vi "Main_Motor_EMG_Control.vi"(0 "VISA Refnum in":refnum<visa-resource-name>, 1 "Motor speed":dbl format="%#_13g", 5 "EMG control":T1(ring)=enum."Biceps contracted", 7 "ID motors":i32[](array[numeric])=[41, 42, 43, 44, 45, 46, 47], 9 "Address current load":u8[](array[numeric])=[108, 110, 112, 114, 116, 118, 120], 11 "error in (no error)":errorcluster, 12 "Old positions":dbl[](array[numeric]), 13 "Old Current (mA)":dbl[](array[numeric])) -> (4 "VISA Refnum out":refnum<visa-resource-name>, 6 "Actual positions":dbl[](array[numeric]), 8 "Current (mA)":dbl[](array[numeric]), 15 "error out":errorcluster)   [LabVIEW 2015]
uses:
  <instrlib>/Dynamixel Motor/Dynamixel Motor.lvlib
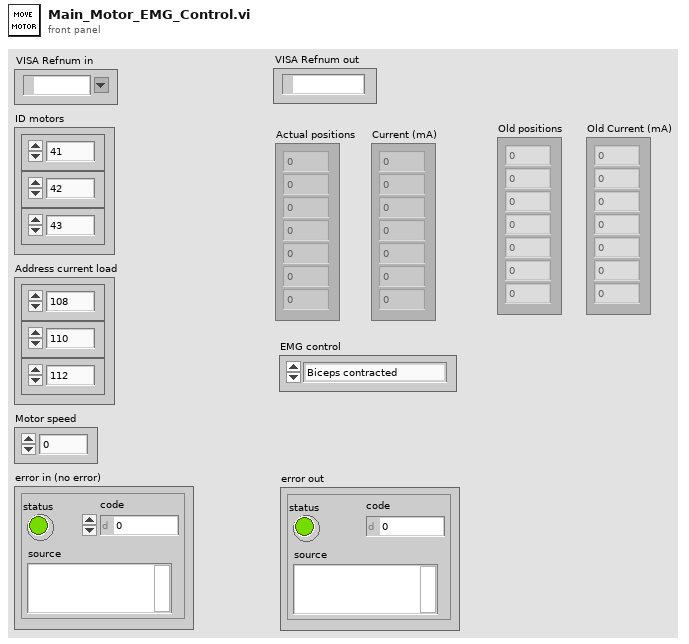
[diagram p1: front panel]
types:
  T1 = enum16{"Biceps contracted M3", "Biceps contracted", "Triceps contracted M3", "Triceps contracted"}
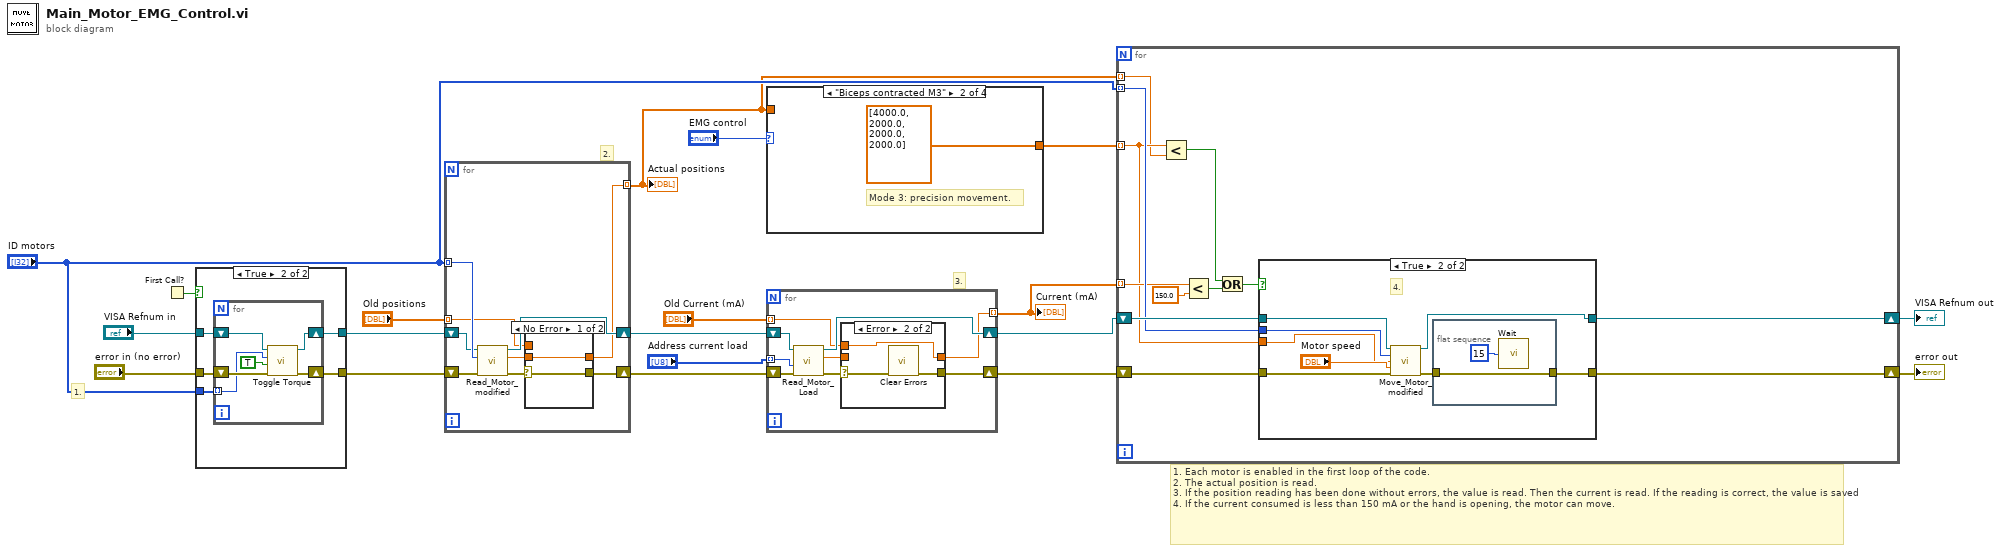
[diagram p0: block diagram]
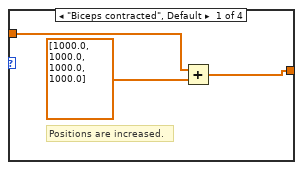
[diagram p2: hidden frame]
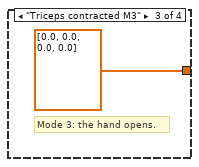
[diagram p3: hidden frame]
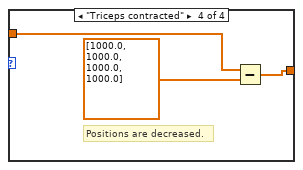
[diagram p4: hidden frame]
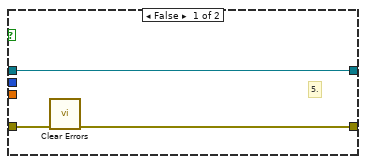
[diagram p5: hidden frame]
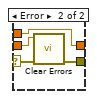
[diagram p7: hidden frame]
diagram:
  # "3."
  # "2."
  # "1."
  # "1. Each motor is enabled in the first loop of the code.\n2. The actual position is read.\n3. If the position reading has been done without errors, the value is read. Then the current is read. If the reading is correct, the value is saved\n4. If the current consumed is less than 150 mA or the hand is opening, the motor can move."
  n1 = First Call?() -> (First Call?: T/F=w10:bool)
  n2 = case shown="True" w10 {
    tunnel: "VISA Refnum in" -> [w20 w26]
    tunnel: "error in (no error)" -> [w21 w25]
    tunnel: [w20 w24] -> w13
    tunnel: [w21 w23] -> w14
    tunnel: "ID motors" -> [_ w22]
    frame False {
    }
    frame True {
      n3 = for {
        shift-right: [w30] -> w24
        shift-left: w26 -> [w31]
        shift-right: [w28] -> w23
        shift-left: w25 -> [w29]
        tunnel: w22 -> [w27] mode=indexing
        n4 = call <instrlib>:"Toggle Torque.vi"("error in (no error)"=w29, "Toggle torque (OFF)"=TRUE, "Motor ID (0)"=w27, "VISA resource name"=w31) -> ("error out"=w28:errorcluster, "VISA resource name out"=w30:refnum<visa-resource-name>)  [unwired: 6 in]
      }
    }
  }
  n5 = for {
    tunnel: "ID motors" -> [w41] mode=indexing
    shift-right: [w33] -> w16
    shift-left: w14 -> [w40]
    shift-right: [w38] -> w15
    shift-left: w13 -> [w39]
    tunnel: [w36] -> w4 mode=indexing
    tunnel: "Old positions" -> [w34] mode=indexing
    n6 = call "Read_Motor_modified.vi"("error in (no error)"=w40, "Motor ID (0)"=w41, "VISA Refnum in"=w39) -> ("error out"=w37:errorcluster, "Position"=w35:dbl, "VISA Refnum out"=w38:refnum<visa-resource-name>)  [unwired: 6 in]
    n7 = case shown="No Error" w37 {
      selector: w37 -> [w42 w45]
      tunnel: [w43 w47] -> w36
      tunnel: w35 -> [w43 w46]
      tunnel: w34 -> [_ w47]
      tunnel: [w42 w44] -> w33
      frame No Error {
      }
      frame Error {
        n8 = call <vilib>:"Clear Errors.vi"("error in (no error)"=w45, "specific error code to clear (0: all)"=w46) -> ("error out"=w44:errorcluster)  [unwired: 4 in, 1 out]
      }
    }
  }
  "Actual positions" <- w4
  n9 = case shown="\"Biceps contracted M3\"" "EMG control" {
    tunnel: w4 -> [w50 _ _ w55]
    tunnel: [w49 dbl[] [4000.0, 2000.0, 2000.0, 2000.0] ("y") dbl[] [0.0, 0.0, 0.0, 0.0] ("y") w53] -> w3
    frame "Biceps contracted", Default {
      # "Positions are increased."
      n10 = Add(x=w50, y=dbl[] [1000.0, 1000.0, 1000.0, 1000.0]) -> (x+y=w49:dbl[])
    }
    frame "Biceps contracted M3" {
      # "Mode 3: precision movement."
    }
    frame "Triceps contracted M3" {
      # "Mode 3: the hand opens."
    }
    frame "Triceps contracted" {
      # "Positions are decreased."
      n11 = Subtract(x=w55, y=dbl[] [1000.0, 1000.0, 1000.0, 1000.0]) -> (x-y=w53:dbl[])
    }
  }
  n12 = for {
    shift-right: [w63] -> w17
    shift-left: w15 -> [w64]
    shift-right: [w56] -> w18
    shift-left: w16 -> [w62]
    tunnel: [w59] -> w19 mode=indexing
    tunnel: "Address current load" -> [w61] mode=indexing
    tunnel: "Old Current (mA)" -> [w58] mode=indexing
    n13 = call "Read_Motor_Load.vi"("error in (no error)"=w62, "Address"=w61, "VISA Refnum in"=w64) -> ("error out"=w57:errorcluster, "Current load"=w60:dbl, "VISA Refnum out"=w63:refnum<visa-resource-name>)  [unwired: 6 in]
    n14 = case shown="Error" w57 {
      selector: w57 -> [w65 w69]
      tunnel: [w66 w67] -> w59
      tunnel: w60 -> [w66 _]
      tunnel: [w65 w68] -> w56
      tunnel: w58 -> [_ w67]
      frame No Error {
      }
      frame Error {
        n15 = call <vilib>:"Clear Errors.vi"("error in (no error)"=w69) -> ("error out"=w68:errorcluster)  [unwired: 5 in, 1 out]
      }
    }
  }
  "Current (mA)" <- w19
  n16 = for {
    shift-right: [w79] -> w6
    shift-left: w17 -> [w81]
    shift-right: [w77] -> w12
    shift-left: w18 -> [w80]
    tunnel: "ID motors" -> [w78] mode=indexing
    tunnel: w3 -> [w71] mode=indexing
    tunnel: w19 -> [w76] mode=indexing
    tunnel: w4 -> [w70] mode=indexing
    n17 = Less?(x=w71, y=w70) -> (x < y?=w74:bool)
    n18 = Less?(x=w76, y=150.0) -> (x < y?=w73:bool)
    n19 = Or(x=w74, y=w73) -> (x .or. y?=w72:bool)
    n20 = case shown="True" w72 {
      tunnel: w81 -> [w83 w92]
      tunnel: w80 -> [w84 w85]
      tunnel: [w83 w91] -> w79
      tunnel: w78 -> [_ w90]
      tunnel: w71 -> [_ w88]
      tunnel: [w82 w86] -> w77
      frame False {
        # "5."
        n21 = call <vilib>:"Clear Errors.vi"("error in (no error)"=w84) -> ("error out"=w82:errorcluster)  [unwired: 5 in, 1 out]
      }
      frame True {
        # "4."
        n22 = call "Move_Motor_modified.vi"("VISA Refnum in"=w92, "Motor ID (0)"=w90, "Goal Position (bit)"=w88, "Goal Speed (RPM)"="Motor speed", "error in (no error)"=w85) -> ("VISA Refnum out"=w91:refnum<visa-resource-name>, "error out"=w87:errorcluster)  [unwired: 9 in]
        n23 = flat-sequence {
          tunnel: [w93] -> w86
          tunnel: w87 -> [w93]
          frame #0 {
            n24 = call "Wait"("Count(mSec)"=u32 15) -> ()  [unwired: 1 out]
          }
        }
      }
    }
  }
  "error out" <- w12
  "VISA Refnum out" <- w6
